vi "Quick Start - Update Channel Metadata.vi"() -> ()   [LabVIEW 2020]
uses:
  channel helper/metadata.ctl
  Nominal Client/Nominal Client.lvclass/Nominal Client.ctl
  dff1568b-51f8-4a1f-98a6-787b133d38ab.vi
  Nominal Client/private_data.set.vi
  <vilib>/Utility/file.llb/Application Directory.vi
  <vilib>/Utility/error.llb/Error Cluster From Error Code.vi
  submodules/reqwest-labview/lv-src/reqwest/create.vi
  Nominal Client/Palette Items/who_am_i.vi
  Nominal Client/asset.get.vi
  User/User.lvclass
  Nominal Client/Nominal Client.lvclass
  nominal types/workspace/workspace.lvclass
  submodules/reqwest-labview/lv-src/reqwest/reqwest.lvclass
  submodules/nominal-streaming-labview-ffi/lv_src/Channel/Channel.lvclass
  submodules/nominal-streaming-labview-ffi/lv_src/Stream/Stream.lvclass
  datasources/dataset/dataset.lvclass
  asset/asset.lvclass
panel:
  out "Updated Metadata":T1
  out "Starting Metadata":T1
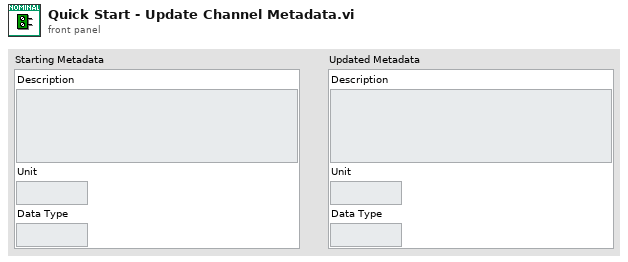
[diagram p1: front panel]
types:
  T1 = typedef "Nominal Client.lvclass/metadata.ctl" = cluster{"Description":string, "Unit":string, "Data Type":string}
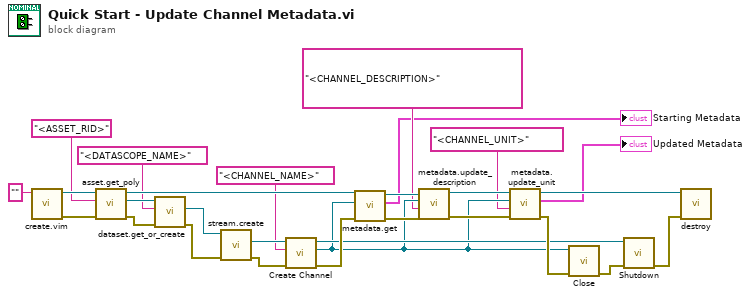
[diagram p0: block diagram]
diagram:
  n1 = call "create.vim"("API Token (string or path)"="") -> ("error out"=w19:errorcluster, "Nominal Client"=w22:refnum<class "Nominal Client.lvclass">)  [unwired: 8 in, 1 out]
  n2 = call-poly "asset.get_poly.vi"("error in"=w19, "Asset RID"="<ASSET_RID>" ("API Token (string or path)"), "Nominal Client in"=w22) -> ("error out"=w16:errorcluster, "Asset"=w20:refnum<class "asset.lvclass">, "Nominal Client out"=w21:refnum<class "Nominal Client.lvclass">)  [unwired: 6 in]
  n3 = call "dataset.get_or_create.vi"("error in"=w16, "Datascope Name"="<DATASCOPE_NAME>" ("API Token (string or path)"), "asset in"=w20) -> ("error out"=w15:errorcluster, "dataset"=w23:refnum<class "dataset.lvclass">)  [unwired: 6 in, 1 out]
  n4 = call "stream.create.vi"("error in (no error)"=w15, "dataset in"=w23) -> ("error out"=w13:errorcluster, "Stream"=w24:refnum<class "Stream.lvclass">)  [unwired: 7 in, 1 out]
  n5 = call "Create Channel.vi"("error in (no error)"=w13, "Channel Name"="<CHANNEL_NAME>", "Nominal Streaming in"=w24) -> ("error out"=w11:errorcluster, "Channel"=w5:refnum<class "Channel.lvclass">, "Nominal Streaming out"=w6:refnum<class "Stream.lvclass">)  [unwired: 6 in]
  n6 = call "metadata.get.vi"("error in"=w11, "Channel"=w5, "Nominal Client in"=w21) -> ("error out"=w10:errorcluster, "Meta Data"=→"Starting Metadata":T1, "Nominal Client out"=w27:refnum<class "Nominal Client.lvclass">)  [unwired: 6 in]
  n7 = call "metadata.update_description.vi"("error in"=w10, "Description"="<CHANNEL_DESCRIPTION>", "Channel"=w5, "Nominal Client in"=w27) -> ("error out"=w9:errorcluster, "Nominal Client out"=w26:refnum<class "Nominal Client.lvclass">)  [unwired: 5 in, 1 out]
  n8 = call "metadata.update_unit.vi"("error in"=w9, "Unit (empty to clear)"="<CHANNEL_UNIT>" ("Description"), "Channel"=w5, "Nominal Client in"=w26) -> ("error out"=w8:errorcluster, "Meta Data"=→"Updated Metadata":T1, "Nominal Client out"=w25:refnum<class "Nominal Client.lvclass">)  [unwired: 5 in]
  n9 = call "Close.vi"("error in (no error)"=w8, "Channel in"=w5) -> ("error out"=w28:errorcluster)  [unwired: 9 in]
  n10 = call "Shutdown.vi"("error in (no error)"=w28, "Nominal Streaming in"=w6) -> ("error out"=w7:errorcluster)  [unwired: 8 in, 1 out]
  n11 = call "destroy.vi"("error in"=w7, "Nominal Client"=w25) -> ()  [unwired: 9 in, 1 out]
